vi "Read.vi"(8 "error in (no error)":errorcluster, 11 "RTFIFODouble in":refnum<class "RTFIFODouble.lvclass">) -> (0 "error out":errorcluster, 1 "timed out?":bool, 2 "Data":dbl, 3 "RTFIFODouble out":refnum<class "RTFIFODouble.lvclass">)   [LabVIEW 2021, in "RTFIFODouble.lvclass"]
uses:
  RTFIFODouble.lvclass
  D:/dev/CIF-LVCore/src/CIFUtilities/CIFChannels/CIFChannels.lvclass
  CIFUtilities/CIFChannels/Typedef/Direction.ctl
  CIFUtilities/CIFChannels/Typedef/Channel State.ctl
  CIFUtilities/CIFChannels/CIFChannels.lvclass/CIFChannels.ctl
  RTFIFODouble.lvclass/RTFIFODouble.ctl
  CIFUtilities/CIFChannels/Accessors/Read Channel State.vi
  CIFUtilities/CIFChannels/Accessors/Read Direction.vi
  CIFUtilities/CIFChannels/CIFChannels.lvclass
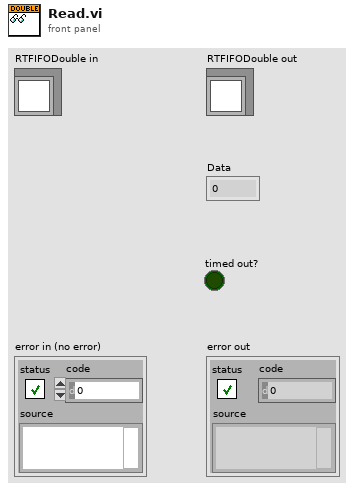
[diagram p1: front panel]
types:
  T1 = typedef "CIFChannels.lvclass/Channel State.ctl" = enum16{"Creating", "Disconnected", "Connecting", "Connected", "Destroying"}
  T2 = typedef "CIFChannels.lvclass/Direction.ctl" = enum16{"Publisher", "Subscriber"}
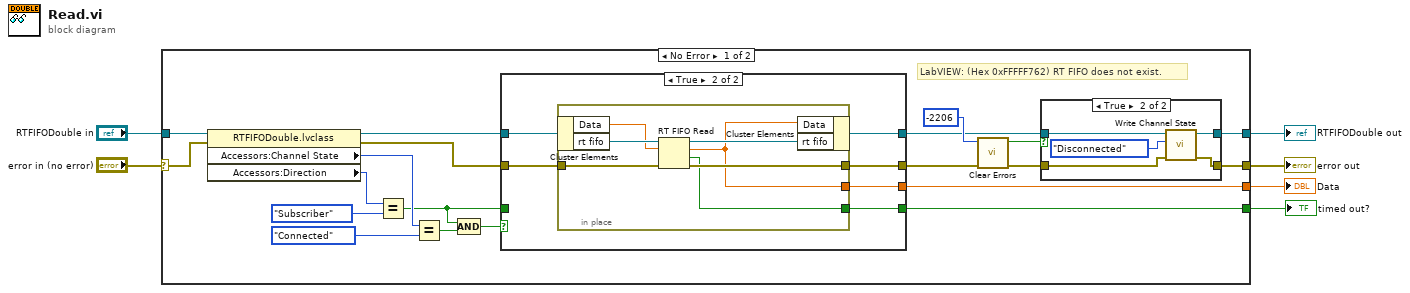
[diagram p0: block diagram]
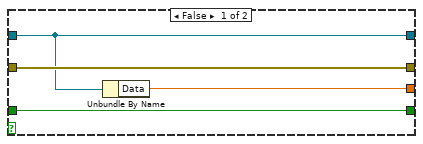
[diagram p3: hidden frame]
diagram:
  n1 = case shown="No Error" "error in (no error)" {
    selector: "error in (no error)" -> [w23 w52]
    tunnel: [w7 w52] -> w5
    tunnel: [w8 w51] -> w3
    tunnel: "RTFIFODouble in" -> [w24 w51]
    tunnel: [w26 _] -> w2
    tunnel: [w25 _] -> w1
    frame No Error {
      # "LabVIEW: (Hex 0xFFFFF762) RT FIFO does not exist."
      n2 = property class="RTFIFODouble.lvclass"(reference=w24, error in=w23) -> (reference out=w22:refnum<class "RTFIFODouble.lvclass">, error out=w21:errorcluster, "Accessors:Channel State"=w18:T1, "Accessors:Direction"=w20:T2)
      n3 = Equal?(x=w20, y=Direction."Subscriber") -> (x = y?=w14:bool)
      n4 = Equal?(x=w18, y=Channel_State."Connected") -> (x = y?=w16:bool)
      n5 = Compound Arithmetic op=AND(w14, w16) -> (w15:bool)
      n6 = case shown="True" w15 {
        tunnel: [w35 w38] -> w10
        tunnel: [w37 w43] -> w12
        tunnel: [w34 w42] -> w26
        tunnel: [w36 w41] -> w25
        tunnel: w21 -> [w37 w40]
        tunnel: w22 -> [w35 w39]
        tunnel: w14 -> [w34 _]
        frame False {
          n7 = Unbundle By Name(w35) -> ("Data"=w36:dbl)
        }
        frame True {
          n8 = in-place {
            in-place-border: w40 -> [w48]
            in-place-border: [w47] -> w43
            in-place-border: [w46] -> w42
            in-place-border: [w44] -> w41
            n9 = in-place-cluster #1(w39) -> ("Data"=w45:dbl, "rt fifo"=w50:refnum<k33>)
            n10 = RT FIFO Read(0:w50, 1:w45, 3:w48) -> (8:w49:refnum<k33>, 9:w44:dbl, 10:w46:bool, 11:w47:errorcluster)  [unwired: 1 in, 1 out]
            n11 = in-place-cluster #1("Data"=w44, "rt fifo"=w49) -> (w38:refnum<class "RTFIFODouble.lvclass">)
          }
        }
      }
      n12 = call <vilib>:"Clear Errors.vi"("error in (no error)"=w12, "specific error code to clear (0: all)"=-2206) -> ("error out"=w9:errorcluster, "specific error cleared?"=w11:bool)  [unwired: 4 in]
      n13 = case shown="True" w11 {
        tunnel: w10 -> [w27 w33]
        tunnel: w9 -> [w28 w32]
        tunnel: [w27 w31] -> w8
        tunnel: [w28 w30] -> w7
        frame False {
        }
        frame True {
          n14 = call "Write Channel State.vi"("error in (no error)"=w32, "Channel State"=Channel_State."Disconnected", "CIFChannels in"=w33) -> ("error out"=w30:errorcluster, "CIFChannels out"=w31:refnum<class "RTFIFODouble.lvclass">)  [unwired: 7 in]
        }
      }
    }
    frame Error {
    }
  }
  "error out" <- w5
  "RTFIFODouble out" <- w3
  "timed out?" <- w2
  "Data" <- w1
